vi "capstone1 ver 4_temp&move code HW code.vi"() -> ()   [LabVIEW 2016]
uses:
  <instrlib>/Dynamixel Motor/Dynamixel Motor.lvlib
  <vilib>/myRIO/Express VI/Onboard Devices/LED/LED Express VI.xnode
  <vilib>/myRIO/Instrument Drivers/Onboard IO/DIO/vis/Write.vi
  <vilib>/myRIO/Instrument Drivers/Onboard IO/DIO/DIO.lvlib
  <vilib>/myRIO/Common/Instrument Driver Framework/myRIO v1.0/DIO/typedefs/DIO Channels Enum.ctl
  <vilib>/myRIO/Common/Instrument Driver Framework/myRIO v1.0/DIO/typedefs/DIO Channels List.ctl
  <vilib>/myRIO/Common/Instrument Driver Framework/Utilities/typedefs/Generic FPGA Reference.ctl
  <vilib>/myRIO/Common/Instrument Driver Framework/Utilities/typedefs/myRIO v1.0 Reference.ctl
  <vilib>/myRIO/Common/Instrument Driver Framework/Utilities/typedefs/Hardware Version Enum.ctl
  <vilib>/myRIO/Common/Instrument Driver Framework/Utilities/typedefs/myRIO Generic Hardware Reference.ctl
  <vilib>/myRIO/Instrument Drivers/Onboard IO/DIO/typedefs/DIO Reference.ctl
  <vilib>/myRIO/Instrument Drivers/Onboard IO/DIO/vis/myRIO DIO Open.xnode
  <vilib>/myRIO/Common/Instrument Driver Framework/Utilities/vis/Is FPGA Ref Available.vi
  <vilib>/myRIO/Common/Instrument Driver Framework/myRIO v1.0/DIO/vis/myRIO v1.1 Open DIO.vi
  <vilib>/userdefined/High Color/nirio_resource_hc.ctl
  <instrlib>/Dynamixel Motor/Public/Motor Operation/Low Level/Baud Setting.ctl
  <vilib>/myRIO/Instrument Drivers/Utilities/Utilities.lvlib
panel:
  out "RT TCP Loop time 4":u32
  out "Numeric":i32
  out "RT TCP Loop time 3":u32
  out "RT TCP Loop time 2":u32
  out "RT TCP Loop time":u32
  out "motor temp":cluster{"0":sgl, "1":sgl, "2":sgl, "3":sgl}
  out "value":T1
  out "TCP Read data":string
  in  "정지":bool
  out "error out":errorcluster
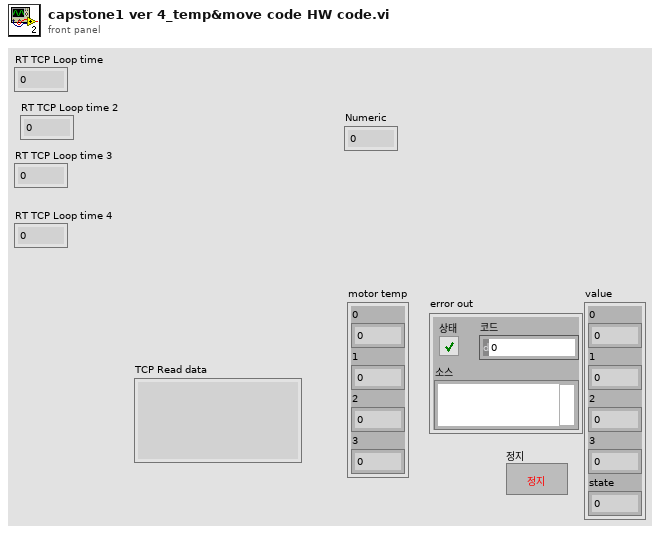
[diagram p1: front panel]
types:
  T1 = cluster{"0":sgl, "1":sgl, "2":sgl, "3":sgl, "state":sgl}
  T2 = typedef "Dynamixel Motor.lvlib/Baud Setting.ctl" = u8
  T3 = enum16{"big-endian, network order", "native, host order", "little-endian"}
  T4 = typedef "DIO.lvlib/DIO Reference.ctl" = cluster{"myRIO Reference":T5, "DIO Channels List":T9}
  T5 = typedef "myRIO Generic Hardware Reference.ctl" = cluster{"myRIO Model":T6, "myRIO Hardware Reference":T7}
  T6 = typedef "Hardware Version Enum.ctl" = enum16{"Unknown", "myRIO-1900", "myRIO-1950", "roboRIO", "NI ELVIS RIO CM"}
  T7 = typedef "myRIO v1.0 Reference.ctl" = cluster{"Generic FPGA Reference":T8, "Allow multiple opens":bool}
  T8 = typedef "Generic FPGA Reference.ctl" = refnum<k20>
  T9 = typedef "DIO Channels List.ctl" = T10[]
  T10 = typedef "DIO Channels Enum.ctl" = enum16{"Not Connected", "C/DIO0", "C/DIO1", "C/DIO2", "C/DIO3", "C/DIO4", "C/DIO5", "C/DIO6", "C/DIO7", "A/DIO0", "A/DIO1", "A/DIO2", "A/DIO3", "A/DIO4", "A/DIO5", "A/DIO6", "A/DIO7", "A/DIO8", "A/DIO9", "A/DIO10", "A/DIO11", "A/DIO12", "A/DIO13", "A/DIO14", "A/DIO15", "B/DIO0", "B/DIO1", "B/DIO2", "B/DIO3", "B/DIO4", "B/DIO5", "B/DIO6", "B/DIO7", "B/DIO8", "B/DIO9", "B/DIO10", "B/DIO11", "B/DIO12", "B/DIO13", "B/DIO14", "B/DIO15", "LED0", "LED1", "LED2", "LED3", "Button0", "DIO/DIO0", "DIO/DIO1", "DIO/DIO2", "DIO/DIO3", "DIO/DIO4", "DIO/DIO5", "DIO/DIO6", "DIO/DIO7", "DIO/DIO8", "DIO/DIO9", "SPI/CS0", "SPI/CS1", "SPI/CS2", "SPI/CS3", "LED RADIO (Green)", "LED RADIO (Red)", "LED COMM (Green)", "LED COMM (Red)", "LED MODE (Green)", "LED MODE (Red)"}
  T11 = typedef "nirio_resource_hc.ctl" = tag
  T12 = cluster{"0":sgl, "1":sgl, "2":sgl, "3":sgl, "state":i32}
  T13 = cluster{"Temperature (C)":u8, "Temperature (C)":u8, "Temperature (C)":u8, "Temperature (C)":u8}
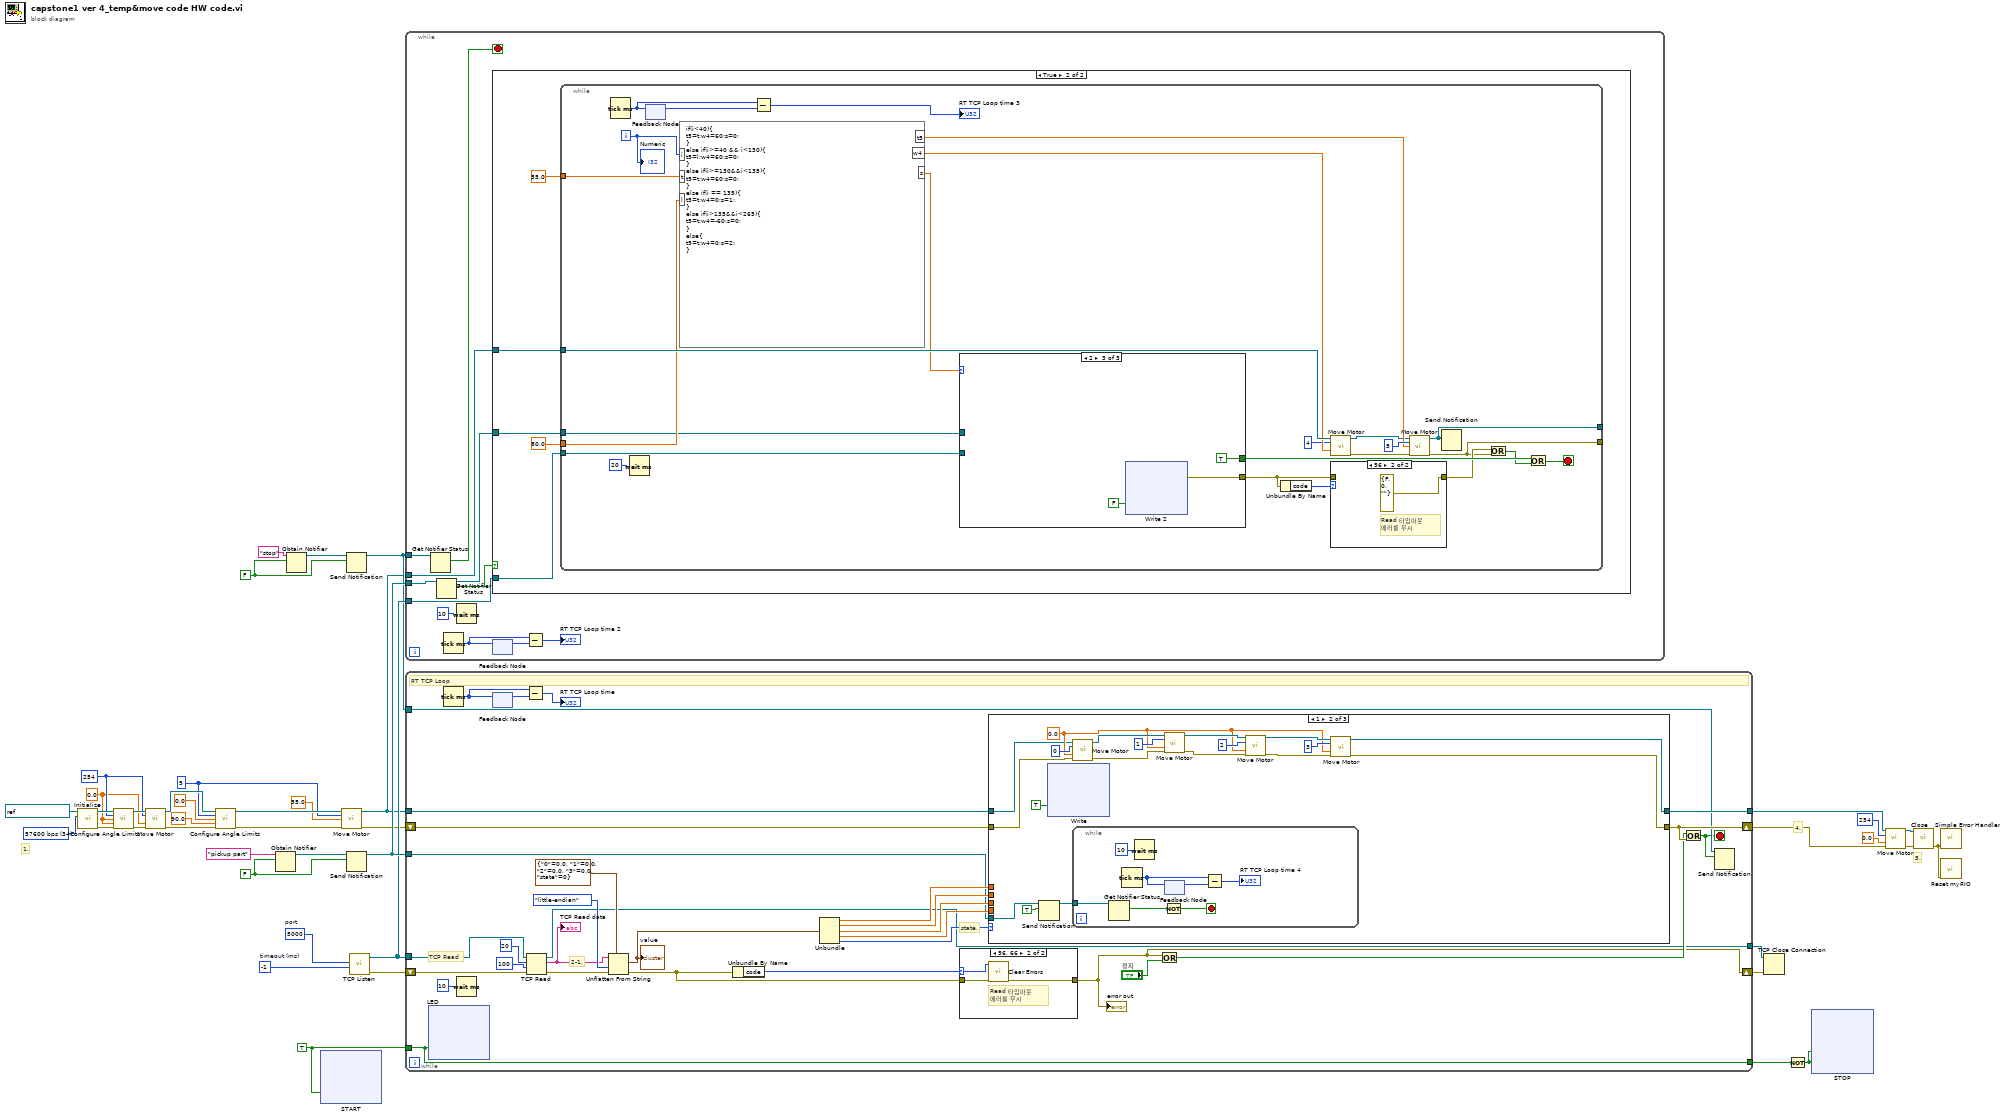
[diagram p0: block diagram]
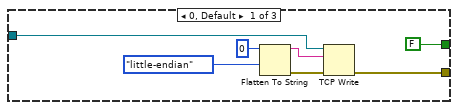
[diagram p4: hidden frame]
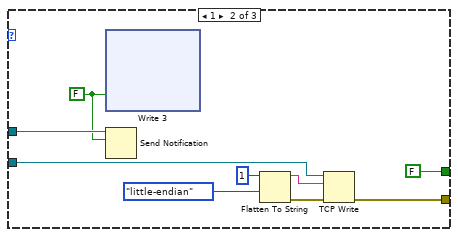
[diagram p5: hidden frame]
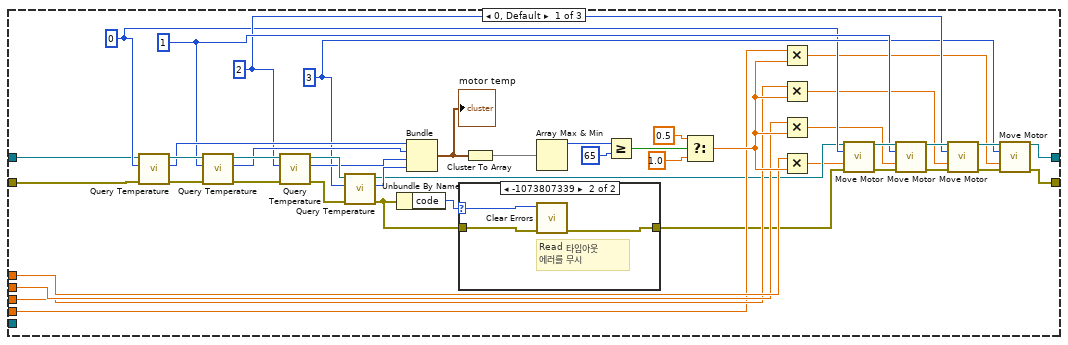
[diagram p6: hidden frame]
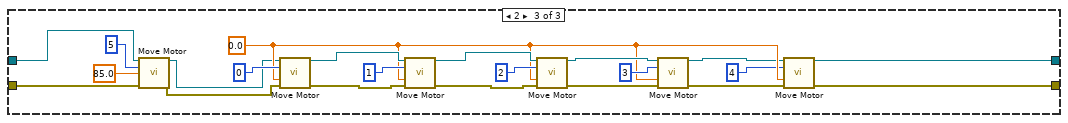
[diagram p8: hidden frame]
diagram:
  w5 = FALSE
  w15 = FALSE
  w8 = 5
  w37 = T2 34 items=["1,000,000 bps"=1, "500,000 bps"=3, "400,000 bps"=4, "250,000 bps"=7, "200,000 bps"=9, "115200 bps"=16, "57600 bps"=34, "19200 bps"=103, "9600 bps"=207] ("Baud rate (57600 bps)")
  w23 = TRUE
  w25 = u8 254 ("Motor ID (0)")
  w24 = 0.0 ("Clockwise Angle Limit (0 deg)")
  w41 = u16 5000  # port
  w42 = -1  # timeout (ms)
  # "5."
  # "4."
  # "1."
  n1 = call <instrlib>:"Initialize.vi"("Baud rate (57600 bps)"=w37, "VISA resource name"=refnum<visa-resource-name> "ASRL3::INSTR") -> ("error out"=w31:errorcluster, "VISA resource name out"=w30:refnum<visa-resource-name>)  [unwired: 8 in]
  n2 = call <instrlib>:"Configure Angle Limits.vi"("VISA resource name"=w30, "Motor ID (0)"=w25, "Clockwise Angle Limit (0 deg)"=w24, "Counter-Clockwise Angle Limit (300 deg)"=w24, "error in (no error)"=w31) -> ("VISA resource name out"=w27:refnum<visa-resource-name>, "error out"=w26:errorcluster)  [unwired: 9 in]
  n3 = call <instrlib>:"Move Motor.vi"("VISA resource name"=w27, "Motor ID (0)"=w25, "Goal Speed (RPM)"=w24, "error in (no error)"=w26) -> ("VISA resource name out"=w21:refnum<visa-resource-name>, "error out"=w22:errorcluster)  [unwired: 10 in]
  n4 = call <instrlib>:"Configure Angle Limits.vi"("VISA resource name"=w21, "Motor ID (0)"=w8, "Clockwise Angle Limit (0 deg)"=0.0, "Counter-Clockwise Angle Limit (300 deg)"=90.0 ("Clockwise Angle Limit (0 deg)"), "error in (no error)"=w22) -> ("VISA resource name out"=w11:refnum<visa-resource-name>, "error out"=w10:errorcluster)  [unwired: 9 in]
  n5 = Obtain Notifier(name (unnamed)="pickup part", notification data type=w15) -> (notifier out=w16:refnum<notifier>)  [unwired: 2 in, 2 out]
  n6 = Obtain Notifier(name (unnamed)="stop", notification data type=w5) -> (notifier out=w6:refnum<notifier>)  [unwired: 2 in, 2 out]
  n7 = xnode "START"("LED0"=w23) -> ()  [unwired: 1 in, 1 out]
  n8 = call <instrlib>:"Move Motor.vi"("VISA resource name"=w11, "Motor ID (0)"=w8, "Goal Position (180 deg)"=55.0, "error in (no error)"=w10) -> ("VISA resource name out"=w1:refnum<visa-resource-name>, "error out"=w9:errorcluster)  [unwired: 10 in]
  n9 = Send Notification(notification=w5, notifier=w6) -> (notifier out=w3:refnum<notifier>)  [unwired: 1 in, 1 out]
  n10 = Send Notification(notification=w15, notifier=w16) -> (notifier out=w14:refnum<notifier>)  [unwired: 1 in, 1 out]
  n11 = call <vilib>:"TCP Listen.vi"("timeout ms (wait forever: -1)"=w42, "port"=w41) -> ("error out"=w38:errorcluster, "connection ID"=w13:refnum<k5>)  [unwired: 5 in, 3 out]
  n12 = while {
    tunnel: w14 -> [w52]
    tunnel: w1 -> [w49]
    tunnel: w13 -> [w48]
    tunnel: w3 -> [w44]
    stop <- w43 stop-if-true
    n13 = Get Notifier Status(notifier=w44) -> (current notification=w43:bool)  [unwired: 1 in, 4 out]
    n14 = Get Notifier Status(notifier=w52) -> (notifier out=w50:refnum<notifier>, current notification=w51:bool)  [unwired: 1 in, 3 out]
    n15 = Tick Count (ms)() -> (millisecond timer value=w46:u32)
    n16 = Wait (ms)(milliseconds to wait=u32 10 ("대기 시간 (ms)")) -> ()  [unwired: 1 out]
    n17 = case shown="True" w51 {
      tunnel: w50 -> [_ w55]
      tunnel: w49 -> [_ w58]
      tunnel: w48 -> [_ w57]
      frame False {
      }
      frame True {
        n18 = while {
          tunnel: w57 -> [w79]
          tunnel: w58 -> [w83]
          tunnel: [w59] -> _
          tunnel: 55.0 -> [w76]
          tunnel: 80.0 -> [w75]
          tunnel: w55 -> [w62]
          tunnel: [w63] -> _
          i -> [w81]
          stop <- w65 stop-if-true
          n19 = Tick Count (ms)() -> (millisecond timer value=w72:u32)
          n20 = Wait (ms)(milliseconds to wait=u32 20 ("대기 시간 (ms)")) -> ()  [unwired: 1 out]
          n21 = feedback #1() -> (w73:u32)  [unwired: 1 in]
          n22 = feedback-in #1(w72) -> ()
          n23 = formula code="if(i<40){\nt5=t;w4=60;s=0;\n}\nelse if(i>=40 && i<130){\nt5=l;w4=60;s=0;\n}\nelse if(i>=130&&i<135){\nt5=t;w4=60;s=0;\n}\nelse if(i == 135){\nt5=t;w4=0;s=1;\n}\nelse if(i>135&&i<265){\nt5=t;w4=-60;s=0;\n}\nelse{\nt5=t;w4=0;s=2;\n}"("i"=w81, "t"=w76, "l"=w75) -> ("t5"=w77:dbl, "w4"=w80:dbl, "s"=w74:dbl)
          n24 = Subtract(x=w72, y=w73) -> (x-y=→"RT TCP Loop time 3":u32)
          n25 = case shown="2" w74 {
            tunnel: w79 -> [w89 w101 _]
            tunnel: w62 -> [_ w97 _]
            tunnel: [FALSE FALSE TRUE] -> w69
            tunnel: [w86 w94 w137] -> w67
            frame 0, Default {
              n26 = Flatten To String(anything=0, byte order (0:big-endian, network order)=T3."little-endian") -> (data string=w90:string, error out=w87:errorcluster)  [unwired: 2 in, 1 out]
              n27 = TCP Write(connection ID=w89, data in=w90, error in (no error)=w87) -> (error out=w86:errorcluster)  [unwired: 1 in, 2 out]
            }
            frame 1 {
              w93 = FALSE ("notification")
              n28 = xnode "Write 3"("LED2"=w93) -> ()  [unwired: 1 in, 1 out]
              n29 = Send Notification(notification=w93, notifier=w97) -> ()  [unwired: 1 in, 2 out]
              n30 = Flatten To String(anything=1, byte order (0:big-endian, network order)=T3."little-endian") -> (data string=w98:string, error out=w95:errorcluster)  [unwired: 2 in, 1 out]
              n31 = TCP Write(connection ID=w101, data in=w98, error in (no error)=w95) -> (error out=w94:errorcluster)  [unwired: 1 in, 2 out]
            }
            frame 2 {
              n32 = xnode "Write 2"("LED2"=FALSE) -> ("error out"=w137:errorcluster)  [unwired: 1 in]
            }
          }
          n33 = Unbundle By Name(w67) -> ("code"=w68:i32)
          n34 = call <instrlib>:"Move Motor.vi"("VISA resource name"=w83, "Motor ID (0)"=4, "Goal Speed (RPM)"=w80) -> ("VISA resource name out"=w61:refnum<visa-resource-name>, "error out"=w70:errorcluster)  [unwired: 11 in]
          n35 = case shown="56" w68 {
            tunnel: [w84 errorcluster {"status"=FALSE, "code"=0, "source"=""} ("에러 출력")] -> w66
            tunnel: w67 -> [w84 _]
            frame 0, Default {
            }
            frame 56 {
              # "Read 타임아웃\n에러를 무시"
            }
          }
          n36 = call <instrlib>:"Move Motor.vi"("VISA resource name"=w61, "Motor ID (0)"=5, "Goal Position (180 deg)"=w77, "error in (no error)"=w70) -> ("VISA resource name out"=w59:refnum<visa-resource-name>, "error out"=w63:errorcluster)  [unwired: 10 in]
          n37 = Send Notification(notification=w59) -> ()  [unwired: 2 in, 2 out]
          n38 = Or(x=w66, y=w63) -> (x .or. y?=w60:bool)
          n39 = Or(x=w69, y=w60) -> (x .or. y?=w65:bool)
          "Numeric" <- w81
        }
      }
    }
    n40 = feedback #2() -> (w47:u32)  [unwired: 1 in]
    n41 = feedback-in #2(w46) -> ()
    n42 = Subtract(x=w46, y=w47) -> (x-y=→"RT TCP Loop time 2":u32)
  }
  n43 = while {
    tunnel: w13 -> [w196]
    tunnel: [w181] -> w40
    shift-right: [w180] -> w39
    shift-left: w38 -> [w197]
    shift-right: [w187] -> w20
    shift-left: w9 -> [w186]
    tunnel: w23 -> [w195]
    tunnel: [w195] -> w33
    tunnel: [w188] -> w19
    tunnel: w14 -> [w179]
    tunnel: w3 -> [w177]
    tunnel: w1 -> [w175]
    stop <- w176 stop-if-true
    # "state."
    # "2-1."
    # "TCP Read"
    # "RT TCP Loop"
    n44 = xnode "LED"("LED1"=w195) -> ()  [unwired: 1 in, 1 out]
    n45 = Tick Count (ms)() -> (millisecond timer value=w183:u32)
    n46 = Wait (ms)(milliseconds to wait=u32 10 ("대기 시간 (ms)")) -> ()  [unwired: 1 out]
    n47 = feedback #3() -> (w184:u32)  [unwired: 1 in]
    n48 = feedback-in #3(w183) -> ()
    n49 = Subtract(x=w183, y=w184) -> (x-y=→"RT TCP Loop time":u32)
    n50 = TCP Read(connection ID=w196, bytes to read=20 ("읽을 바이트"), error in (no error)=w197, 9:100 ("타임아웃 ms (25000)")) -> (connection ID out=w181:refnum<k5>, data out=w200:string, error out=w199:errorcluster)  [unwired: 1 in]
    "TCP Read data" <- w200
    n51 = Unflatten From String(type=T12 {"0"=0.0, "1"=0.0, "2"=0.0, "3"=0.0, "state"=0}, binary string=w200, byte order (0:big-endian, network order)=T3."little-endian", error in (no error)=w199) -> (value=w194:T12, error out=w198:errorcluster)  [unwired: 1 in, 1 out]
    "value" <- w194
    n52 = Unbundle By Name(w198) -> ("code"=w205:i32)
    n53 = Unbundle(w194) -> ("0"=w193:sgl, "1"=w191:sgl, "2"=w192:sgl, "3"=w190:sgl, "state"=w189:i32)
    n54 = case shown="56, 66" w205 {
      selector: w205 -> [_ w375]
      tunnel: [w373 w374] -> w180
      tunnel: w198 -> [w373 w376]
      frame 0, Default {
      }
      frame 56, 66 {
        # "Read 타임아웃\n에러를 무시"
        n55 = call <vilib>:"Clear Errors.vi"("error in (no error)"=w376, "specific error code to clear (0: all)"=w375) -> ("error out"=w374:errorcluster)  [unwired: 4 in, 1 out]
      }
    }
    "error out" <- w180
    n56 = case shown="1" w189 {
      tunnel: w193 -> [w234 _ _]
      tunnel: w191 -> [w233 _ _]
      tunnel: w192 -> [w232 _ _]
      tunnel: w190 -> [w231 _ _]
      tunnel: [w216 w261 w324] -> w188
      tunnel: [w217 w260 w323] -> w187
      tunnel: w186 -> [w214 w262 w320]
      tunnel: w179 -> [_ w259 _]
      tunnel: w175 -> [w207 w255 w316]
      frame 0, Default {
        w218 = 3
        w219 = 2
        w220 = 1
        w215 = 0
        n57 = call <instrlib>:"Query Temperature.vi"("error in"=w214, "Motor ID (0)"=w215, "VISA resource name"=w207) -> ("error out"=w241:errorcluster, "Temperature (C)"=w230:u8, "VISA resource name out"=w244:refnum<visa-resource-name>)  [unwired: 6 in]
        n58 = call <instrlib>:"Query Temperature.vi"("error in"=w241, "Motor ID (0)"=w220, "VISA resource name"=w244) -> ("error out"=w240:errorcluster, "Temperature (C)"=w229:u8, "VISA resource name out"=w243:refnum<visa-resource-name>)  [unwired: 6 in]
        n59 = call <instrlib>:"Query Temperature.vi"("error in"=w240, "Motor ID (0)"=w219, "VISA resource name"=w243) -> ("error out"=w239:errorcluster, "Temperature (C)"=w228:u8, "VISA resource name out"=w242:refnum<visa-resource-name>)  [unwired: 6 in]
        n60 = call <instrlib>:"Query Temperature.vi"("error in"=w239, "Motor ID (0)"=w218, "VISA resource name"=w242) -> ("error out"=w221:errorcluster, "Temperature (C)"=w227:u8, "VISA resource name out"=w213:refnum<visa-resource-name>)  [unwired: 6 in]
        n61 = Unbundle By Name(w221) -> ("code"=w222:i32)
        n62 = Bundle("Temperature (C)"=w230, "Temperature (C)"=w229, "Temperature (C)"=w228, "Temperature (C)"=w227) -> (w224:T13)  [unwired: 1 in]
        "motor temp" <- w224
        n63 = case shown="-1073807339" w222 {
          selector: w222 -> [_ w253]
          tunnel: [w251 w252] -> w212
          tunnel: w221 -> [w251 w254]
          frame 0, Default {
          }
          frame -1073807339 {
            # "Read 타임아웃\n에러를 무시"
            n64 = call <vilib>:"Clear Errors.vi"("error in (no error)"=w254, "specific error code to clear (0: all)"=w253) -> ("error out"=w252:errorcluster)  [unwired: 4 in, 1 out]
          }
        }
        n65 = Cluster To Array(cluster=w224) -> (array=w226:u8[])
        n66 = Array Max & Min(array=w226) -> (max value=w225:u8)  [unwired: 3 out]
        n67 = Greater Or Equal?(x=w225, y=65) -> (x >= y?=w223:bool)
        n68 = Select(t=0.5, s=w223, f=1.0) -> (s? t:f=w235:dbl)
        n69 = Multiply(x=w231, y=w235) -> (x*y=w208:dbl)
        n70 = Multiply(x=w232, y=w235) -> (x*y=w209:dbl)
        n71 = Multiply(x=w233, y=w235) -> (x*y=w210:dbl)
        n72 = Multiply(x=w234, y=w235) -> (x*y=w211:dbl)
        n73 = call <instrlib>:"Move Motor.vi"("VISA resource name"=w213, "Motor ID (0)"=w215, "Goal Speed (RPM)"=w211, "error in (no error)"=w212) -> ("VISA resource name out"=w245:refnum<visa-resource-name>, "error out"=w246:errorcluster)  [unwired: 10 in]
        n74 = call <instrlib>:"Move Motor.vi"("VISA resource name"=w245, "Motor ID (0)"=w220, "Goal Speed (RPM)"=w210, "error in (no error)"=w246) -> ("VISA resource name out"=w247:refnum<visa-resource-name>, "error out"=w249:errorcluster)  [unwired: 10 in]
        n75 = call <instrlib>:"Move Motor.vi"("VISA resource name"=w247, "Motor ID (0)"=w219, "Goal Speed (RPM)"=w209, "error in (no error)"=w249) -> ("VISA resource name out"=w248:refnum<visa-resource-name>, "error out"=w250:errorcluster)  [unwired: 10 in]
        n76 = call <instrlib>:"Move Motor.vi"("VISA resource name"=w248, "Motor ID (0)"=w218, "Goal Speed (RPM)"=w208, "error in (no error)"=w250) -> ("VISA resource name out"=w216:refnum<visa-resource-name>, "error out"=w217:errorcluster)  [unwired: 10 in]
      }
      frame 1 {
        w263 = 0.0
        n77 = Send Notification(notification=TRUE, notifier=w259) -> (notifier out=w257:refnum<notifier>)  [unwired: 1 in, 1 out]
        n78 = xnode "Write"("LED2"=TRUE) -> ()  [unwired: 1 in, 1 out]
        n79 = call <instrlib>:"Move Motor.vi"("VISA resource name"=w255, "Motor ID (0)"=0, "Goal Speed (RPM)"=w263, "error in (no error)"=w262) -> ("VISA resource name out"=w264:refnum<visa-resource-name>, "error out"=w265:errorcluster)  [unwired: 10 in]
        n80 = while {
          tunnel: w257 -> [w314]
          stop <- w312 stop-if-true
          n81 = Get Notifier Status(notifier=w314) -> (current notification=w313:bool)  [unwired: 1 in, 4 out]
          n82 = Tick Count (ms)() -> (millisecond timer value=w309:u32)
          n83 = Wait (ms)(milliseconds to wait=u32 10 ("대기 시간 (ms)")) -> ()  [unwired: 1 out]
          n84 = Not(x=w313) -> (.not. x?=w312:bool)
          n85 = feedback #4() -> (w311:u32)  [unwired: 1 in]
          n86 = feedback-in #4(w309) -> ()
          n87 = Subtract(x=w309, y=w311) -> (x-y=→"RT TCP Loop time 4":u32)
        }
        n88 = call <instrlib>:"Move Motor.vi"("VISA resource name"=w264, "Motor ID (0)"=1, "Goal Speed (RPM)"=w263, "error in (no error)"=w265) -> ("VISA resource name out"=w266:refnum<visa-resource-name>, "error out"=w268:errorcluster)  [unwired: 10 in]
        n89 = call <instrlib>:"Move Motor.vi"("VISA resource name"=w266, "Motor ID (0)"=2, "Goal Speed (RPM)"=w263, "error in (no error)"=w268) -> ("VISA resource name out"=w267:refnum<visa-resource-name>, "error out"=w269:errorcluster)  [unwired: 10 in]
        n90 = call <instrlib>:"Move Motor.vi"("VISA resource name"=w267, "Motor ID (0)"=3, "Goal Speed (RPM)"=w263, "error in (no error)"=w269) -> ("VISA resource name out"=w261:refnum<visa-resource-name>, "error out"=w260:errorcluster)  [unwired: 10 in]
      }
      frame 2 {
        w327 = 0.0
        n91 = call <instrlib>:"Move Motor.vi"("VISA resource name"=w316, "Motor ID (0)"=5, "Goal Position (180 deg)"=85.0, "error in (no error)"=w320) -> ("VISA resource name out"=w318:refnum<visa-resource-name>, "error out"=w319:errorcluster)  [unwired: 10 in]
        n92 = call <instrlib>:"Move Motor.vi"("VISA resource name"=w318, "Motor ID (0)"=0, "Goal Speed (RPM)"=w327, "error in (no error)"=w319) -> ("VISA resource name out"=w337:refnum<visa-resource-name>, "error out"=w336:errorcluster)  [unwired: 10 in]
        n93 = call <instrlib>:"Move Motor.vi"("VISA resource name"=w337, "Motor ID (0)"=1, "Goal Speed (RPM)"=w327, "error in (no error)"=w336) -> ("VISA resource name out"=w335:refnum<visa-resource-name>, "error out"=w333:errorcluster)  [unwired: 10 in]
        n94 = call <instrlib>:"Move Motor.vi"("VISA resource name"=w335, "Motor ID (0)"=2, "Goal Speed (RPM)"=w327, "error in (no error)"=w333) -> ("VISA resource name out"=w334:refnum<visa-resource-name>, "error out"=w332:errorcluster)  [unwired: 10 in]
        n95 = call <instrlib>:"Move Motor.vi"("VISA resource name"=w334, "Motor ID (0)"=3, "Goal Speed (RPM)"=w327, "error in (no error)"=w332) -> ("VISA resource name out"=w325:refnum<visa-resource-name>, "error out"=w322:errorcluster)  [unwired: 10 in]
        n96 = call <instrlib>:"Move Motor.vi"("VISA resource name"=w325, "Motor ID (0)"=4, "Goal Speed (RPM)"=w327, "error in (no error)"=w322) -> ("VISA resource name out"=w324:refnum<visa-resource-name>, "error out"=w323:errorcluster)  [unwired: 10 in]
      }
    }
    n97 = Or(x=w180, y="정지") -> (x .or. y?=w185:bool)
    n98 = Or(x=w185, y=w187) -> (x .or. y?=w176:bool)
    n99 = Send Notification(notification=w176, notifier=w177) -> ()  [unwired: 1 in, 2 out]
  }
  n100 = TCP Close Connection(connection ID=w40, error in (no error)=w39) -> ()  [unwired: 3 out]
  n101 = Not(x=w33) -> (.not. x?=w32:bool)
  n102 = xnode "STOP"("LED0"=w32, "LED1"=w32) -> ()  [unwired: 1 in, 1 out]
  n103 = call <instrlib>:"Move Motor.vi"("VISA resource name"=w19, "Motor ID (0)"=u8 254, "Goal Speed (RPM)"=0.0, "error in (no error)"=w20) -> ("VISA resource name out"=w18:refnum<visa-resource-name>, "error out"=w17:errorcluster)  [unwired: 10 in]
  n104 = call <instrlib>:"Close.vi"("error in (no error)"=w17, "VISA resource name"=w18) -> ("error out"=w2:errorcluster)  [unwired: 9 in]
  n105 = call <vilib>:"Simple Error Handler.vi"("error in (no error)"=w2) -> ()  [unwired: 4 in, 5 out]
  n106 = call <vilib>:"Reset myRIO.vi"("error in (no error)"=w2) -> ()  [unwired: 10 in, 1 out]
